vi "MeanOfArray (SubVI).vi"(11 "Array":dbl[](array[numeric])) -> (3 "Mean":dbl)   [LabVIEW 2015]
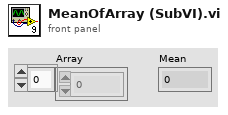
[diagram p1: front panel]
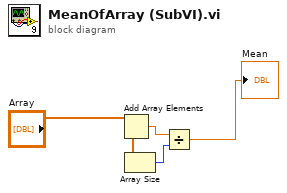
[diagram p0: block diagram]
diagram:
  n1 = Add Array Elements(numeric array="Array") -> (sum=w1:dbl)
  n2 = Array Size(array="Array") -> (size(s)=w2:i32)
  n3 = Divide(x=w1, y=w2) -> (x/y=→"Mean":dbl)
